vi "Interpolate_Calib_Coeff.vi"(5 "Analysis Info cluster":T1={"Colour"=0, "Inst type"=enum."Pitot-static tube", "Inst name"="Manometer voltage", "Symbol"="U", "Code name"="", "Extra Info"="U", "Inst Array"=enum."PWA", "Extra Titles"=[], "Extra Values"=[], "U"=0.0, "u^2"=0.0, "u^3"=0.0, "u^4"=0.0, "Skew_u"=0.0, "Kurt_u"=0.0, "Sd Error in Mean"=0.0, "% u'/U"=0.0, "X"=0.0, "Y"=0.0, "Z"=0.0, "Timescale integral to 25%"=0.0, "Sd Error in Variance"=0.0, "Calib File"=path "", "Calib Constants"=[], "Output Position"=FALSE, "Full Stats"=FALSE, "Av Sampling Rate"=0.0, "Av No of Samples"=0.0, "Total Meas Time (s)"=0.0, "ADAM Ch Name"=""} {"Sd Error in Variance" format="%.2f"; "Skew_u" format="%.2f"; "% u'/U" format="%.2f"; "Sd Error in Mean" format="%.2f"; "Kurt_u" format="%.2f"; "u^4" format="%.2f"; "u^3" format="%.2f"; "U" format="%.2f"; "u^2" format="%.2f"}, 7 "Take New Data?":bool) -> (0 "Calib Coeff":dbl[](array[numeric]), 1 "Calib Type Name":string, 2 "Calib file string":string, 3 "Read file":bool, 4 "Analysis Info cluster  Out":T1={"Colour"=0, "Inst type"=enum."Pitot-static tube", "Inst name"="Manometer voltage", "Symbol"="U", "Code name"="", "Extra Info"="U", "Inst Array"=enum."PWA", "Extra Titles"=[], "Extra Values"=[], "U"=0.0, "u^2"=0.0, "u^3"=0.0, "u^4"=0.0, "Skew_u"=0.0, "Kurt_u"=0.0, "Sd Error in Mean"=0.0, "% u'/U"=0.0, "X"=0.0, "Y"=0.0, "Z"=0.0, "Timescale integral to 25%"=0.0, "Sd Error in Variance"=0.0, "Calib File"=path "", "Calib Constants"=[], "Output Position"=FALSE, "Full Stats"=FALSE, "Av Sampling Rate"=0.0, "Av No of Samples"=0.0, "Total Meas Time (s)"=0.0, "ADAM Ch Name"=""} {"Sd Error in Variance" format="%.2f"; "Skew_u" format="%.2f"; "% u'/U" format="%.2f"; "Sd Error in Mean" format="%.2f"; "Kurt_u" format="%.2f"; "u^4" format="%.2f"; "u^3" format="%.2f"; "U" format="%.2f"; "u^2" format="%.2f"})   [LabVIEW 2012]
uses:
  Controls/Analysis_info_cluster.ctl
  Controls/Inst_type.ctl
  Controls/Instrument_Array.ctl
  XW calib map/Map method.ctl
  Globals/Meas_global.vi
  XW calib map/XW_Map_Global.vi
  Globals/Plug_in_data_global.vi
  <vilib>/Analysis/NI_AALPro.lvlib
panel:
  in  "TAKE NEW DATA XW Map method":T4=enum."Const. Psi_eff (std.)"
  in  "Domain padding factor":dbl=1.01
  in  "cap indicial sum to n":bool=TRUE
  in  "surface order (n)":i32=5
  in  "Apply calibration corrections":bool=TRUE
  in  "POST PROC. XW Map method":T4=enum."Psi_eff, k = f(Umagn.)"
  in  "variable n":bool=TRUE
  in  "wire diameter (mu.m)":dbl=5.0
  out "Header info":string[][](array[string])
  # "For polysurface method only:"
  # "For trimesh method only"
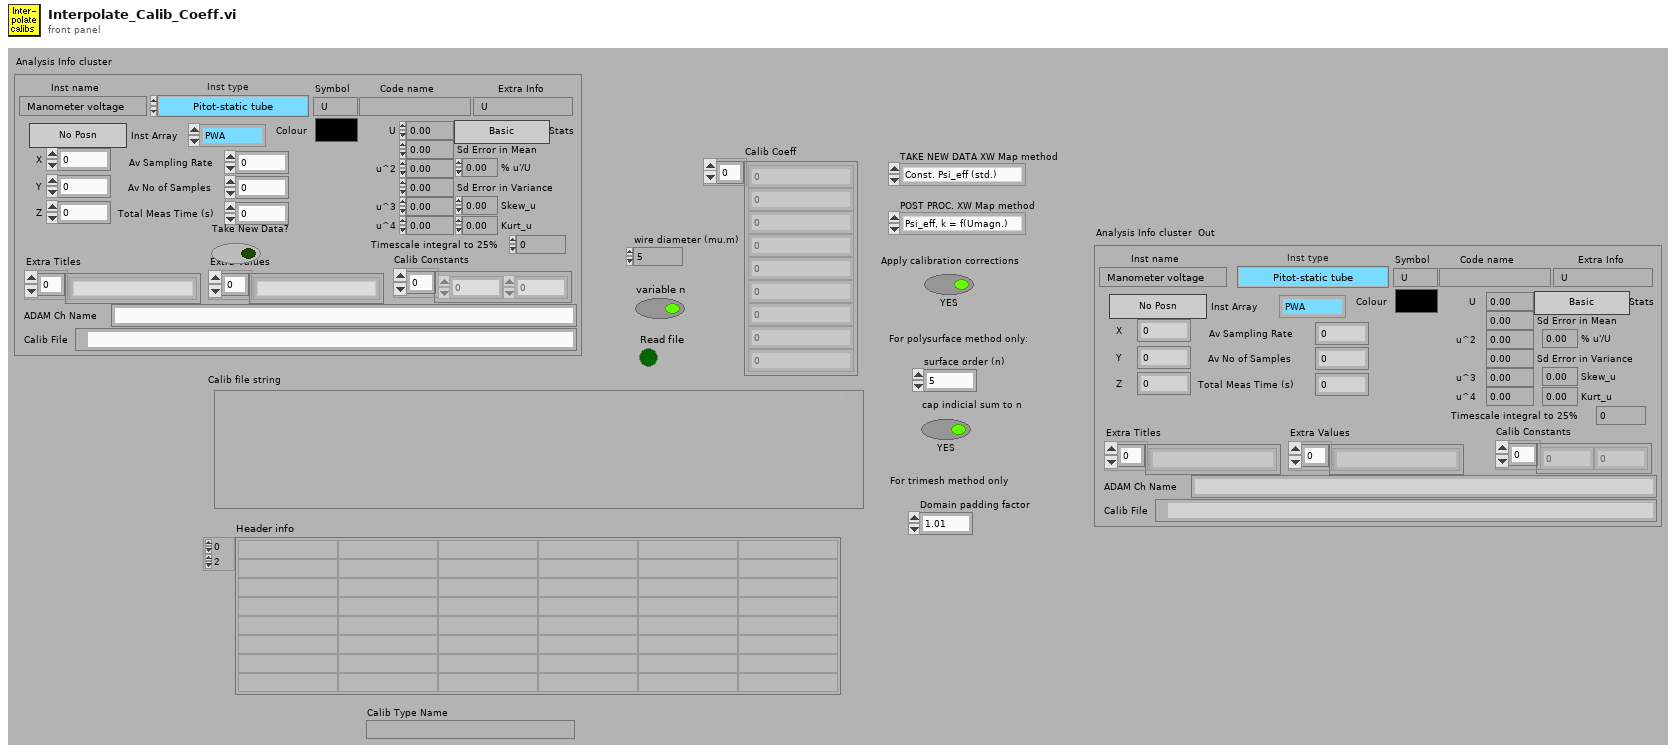
[diagram p1: front panel]
types:
  T1 = typedef "Analysis_info_cluster.ctl" = cluster{"Colour":u32, "Inst type":T2, "Inst name":string, "Symbol":string, "Code name":string, "Extra Info":string, "Inst Array":T3, "Extra Titles":string[], "Extra Values":string[], "U":dbl, "u^2":dbl, "u^3":dbl, "u^4":dbl, "Skew_u":dbl, "Kurt_u":dbl, "Sd Error in Mean":dbl, "% u'/U":dbl, "X":dbl, "Y":dbl, "Z":dbl, "Timescale integral to 25%":dbl, "Sd Error in Variance":dbl, "Calib File":path, "Calib Constants":dbl[], "Output Position":bool, "Full Stats":bool, "Av Sampling Rate":dbl, "Av No of Samples":dbl, "Total Meas Time (s)":dbl, "ADAM Ch Name":string}
  T2 = typedef "Inst_type.ctl" = enum16{"Propeller anemometer", "Raw voltage", "Pressure Transducer", "Pitot-static tube", "Preston tube", "Hot wire", "Cross wire 1", "Cross wire 2", "Generic Linear", "Generic Polynomial", "Generic BackPoly", "Fast FID", "Thermocouple", "Cold wire", "Pulsed Wire", "LDA Vel", "LDA Tran time", "LDA Arr time"}
  T3 = typedef "Instrument_Array.ctl" = enum16{"PWA", "LDA", "Analogue"}
  T4 = typedef "Map method.ctl" = enum16{"Triangle mesh", "Polynomial surface", "Const. Psi_eff (std.)", "Psi_eff = f(Umagn.)", "Psi_eff, k = f(Umagn.)"}
  T5 = cluster{"1st Calib time":dbl, "2nd Calib time":dbl, "Meas start time":dbl, "Meas end time":dbl, "Fraction":dbl}
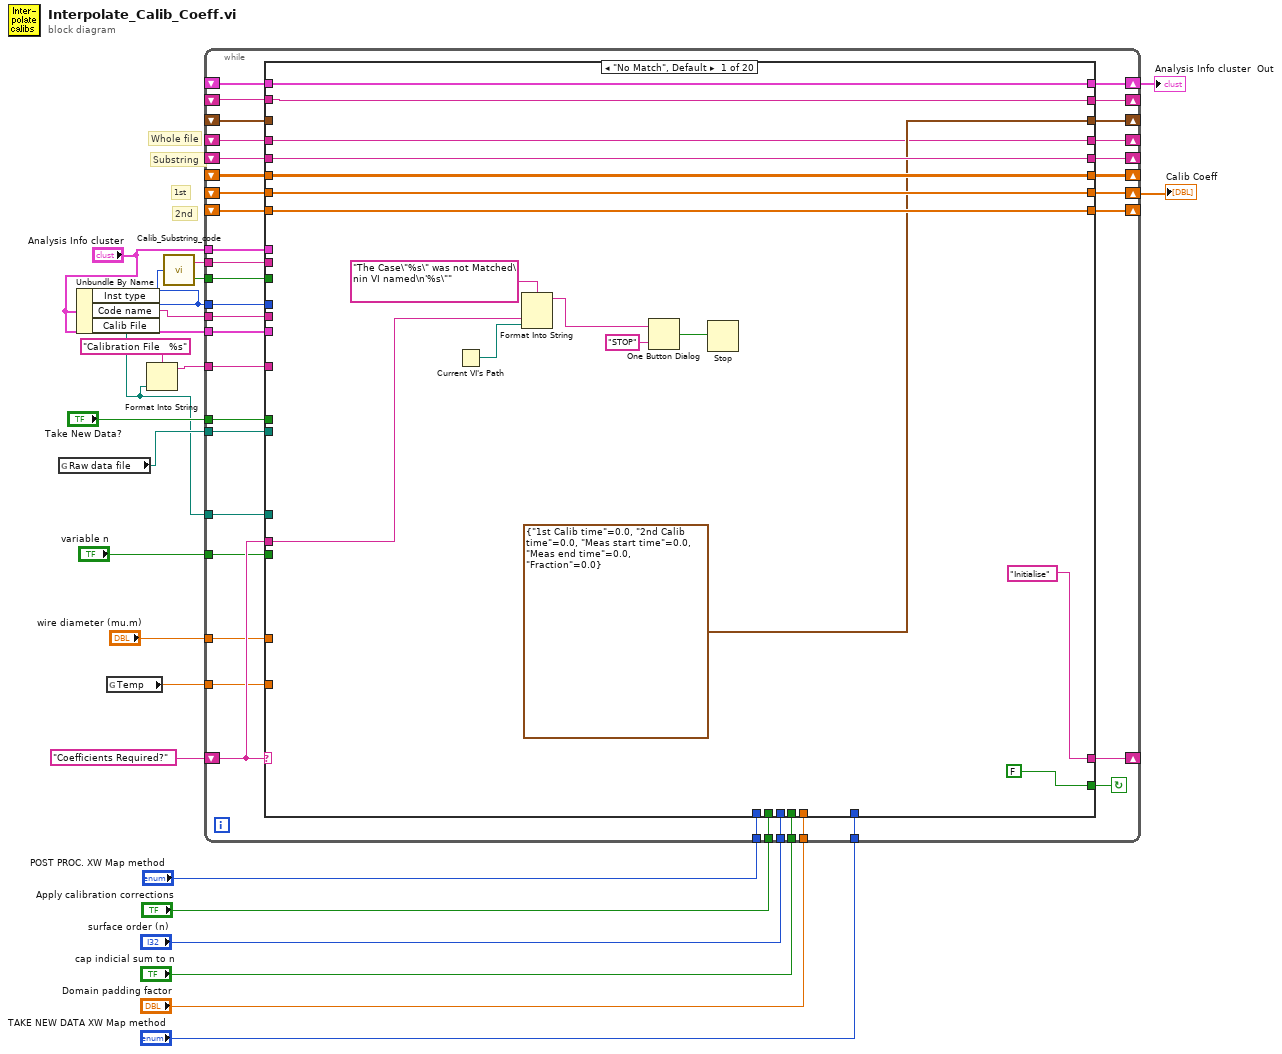
[diagram p0: block diagram]
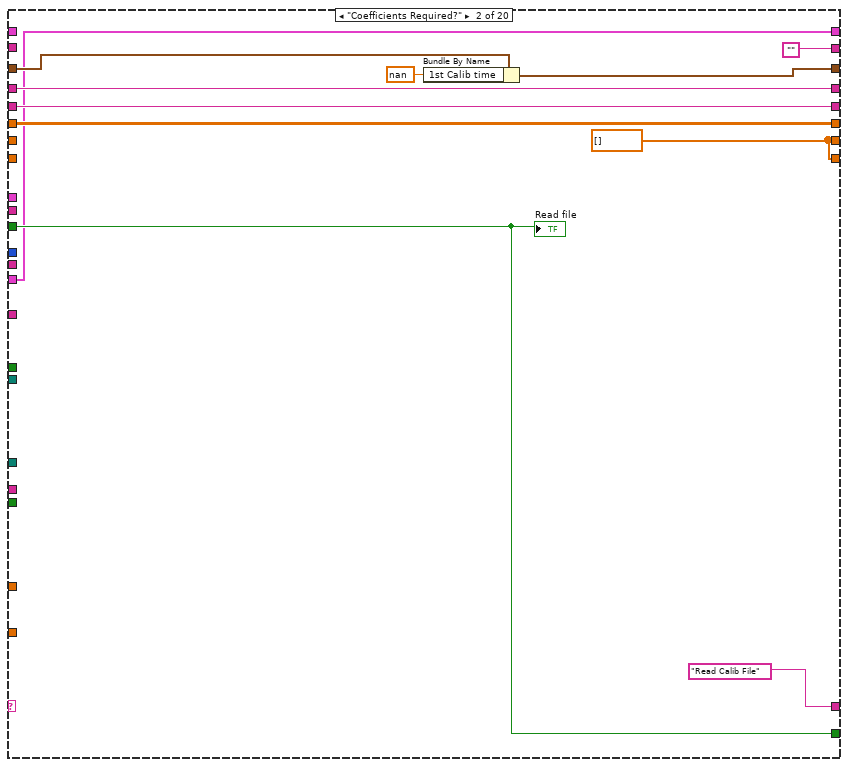
[diagram p2: hidden frame]
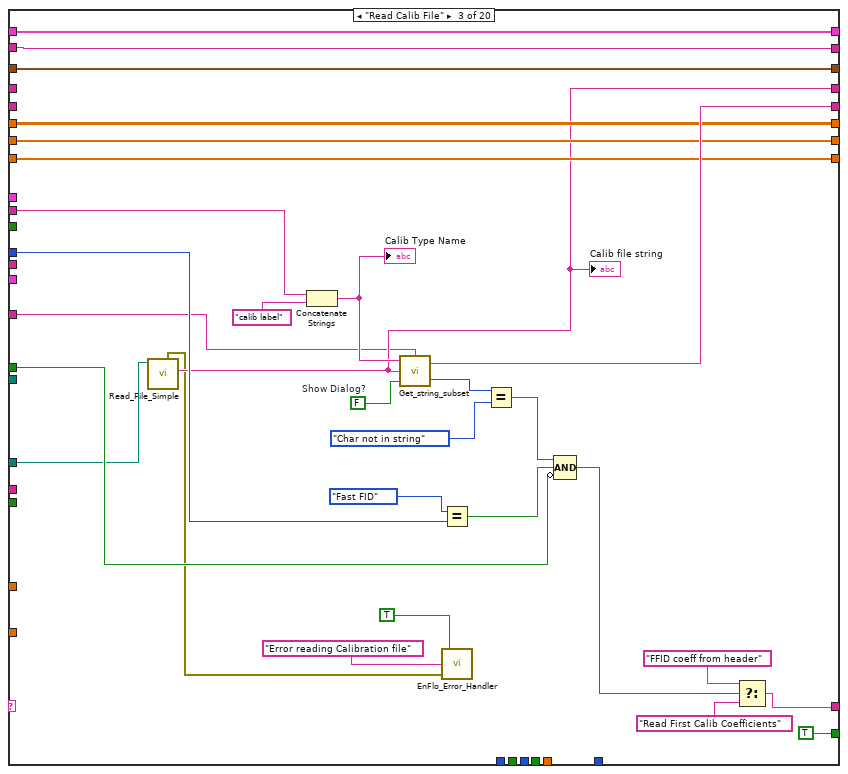
[diagram p3: hidden frame]
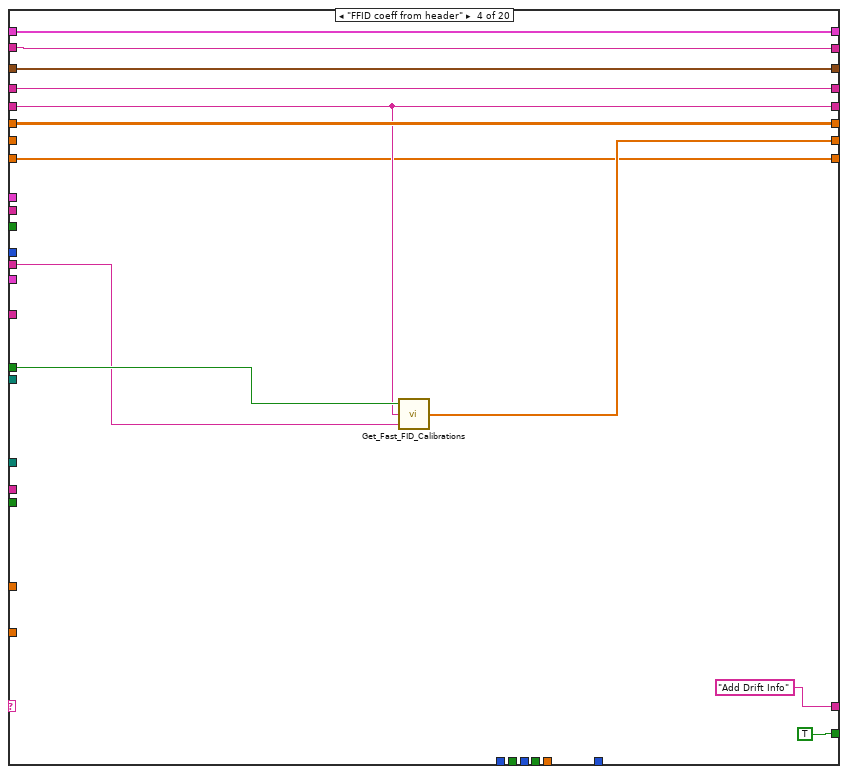
[diagram p4: hidden frame]
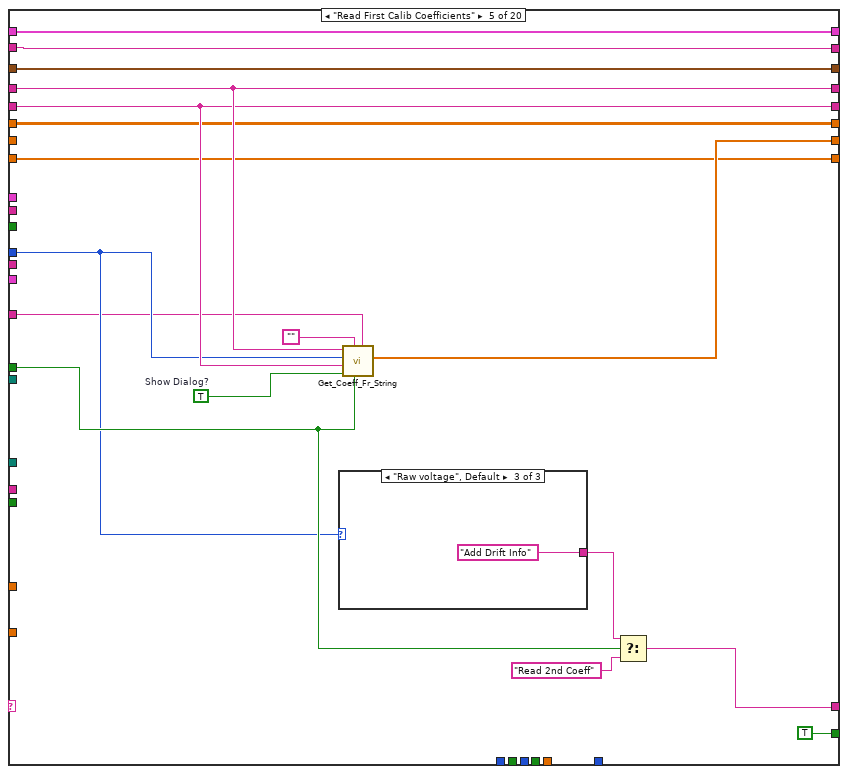
[diagram p5: hidden frame]
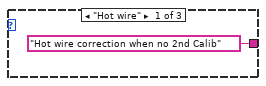
[diagram p6: hidden frame]
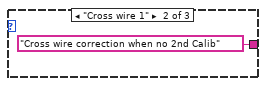
[diagram p7: hidden frame]
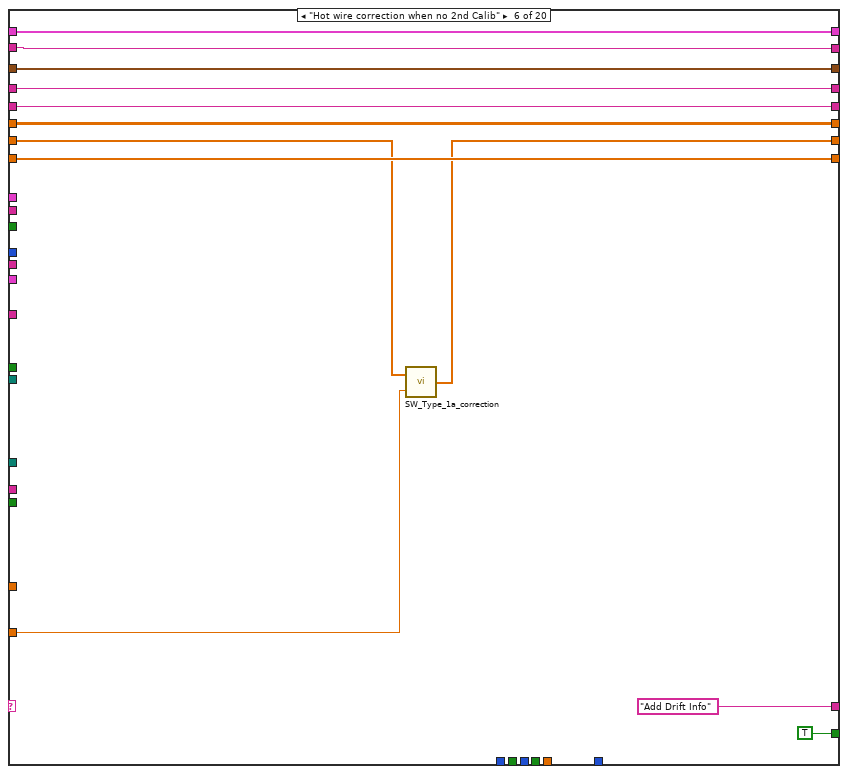
[diagram p8: hidden frame]
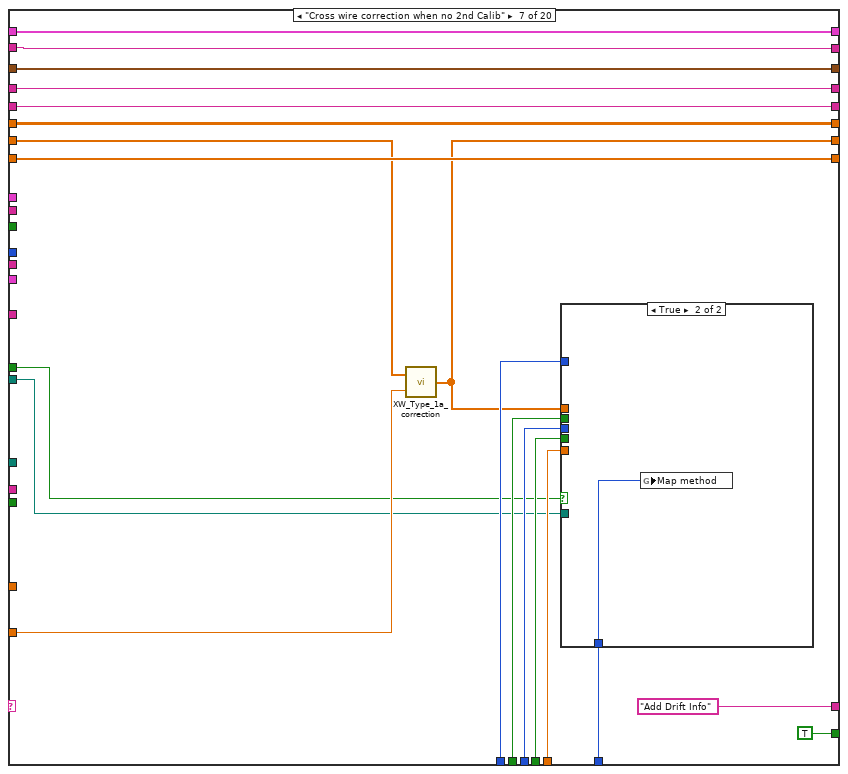
[diagram p9: hidden frame]
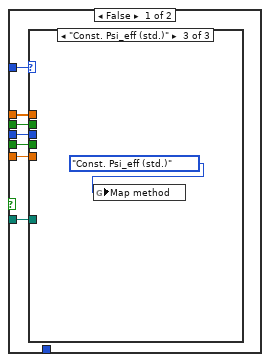
[diagram p10: hidden frame]
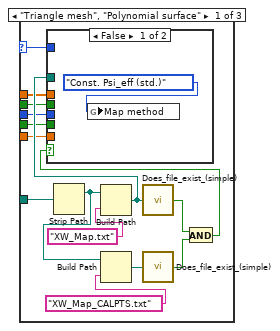
[diagram p11: hidden frame]
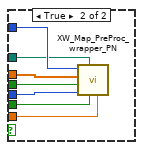
[diagram p12: hidden frame]
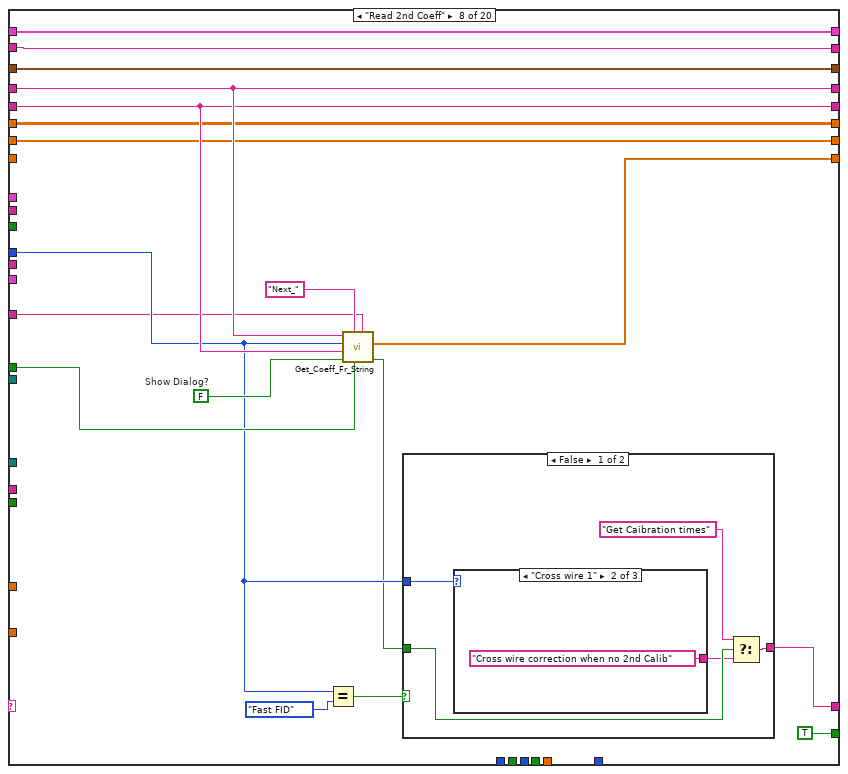
[diagram p14: hidden frame]
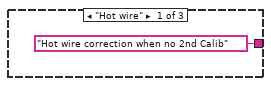
[diagram p15: hidden frame]
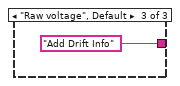
[diagram p16: hidden frame]
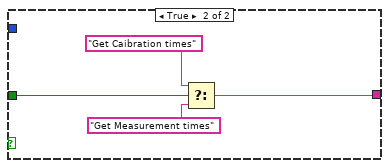
[diagram p17: hidden frame]
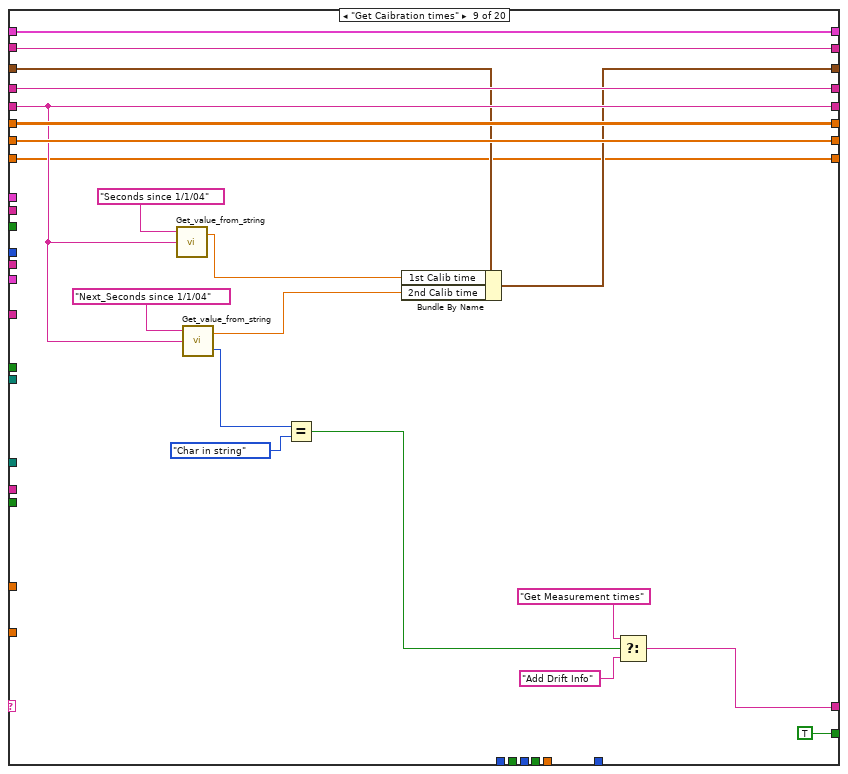
[diagram p18: hidden frame]
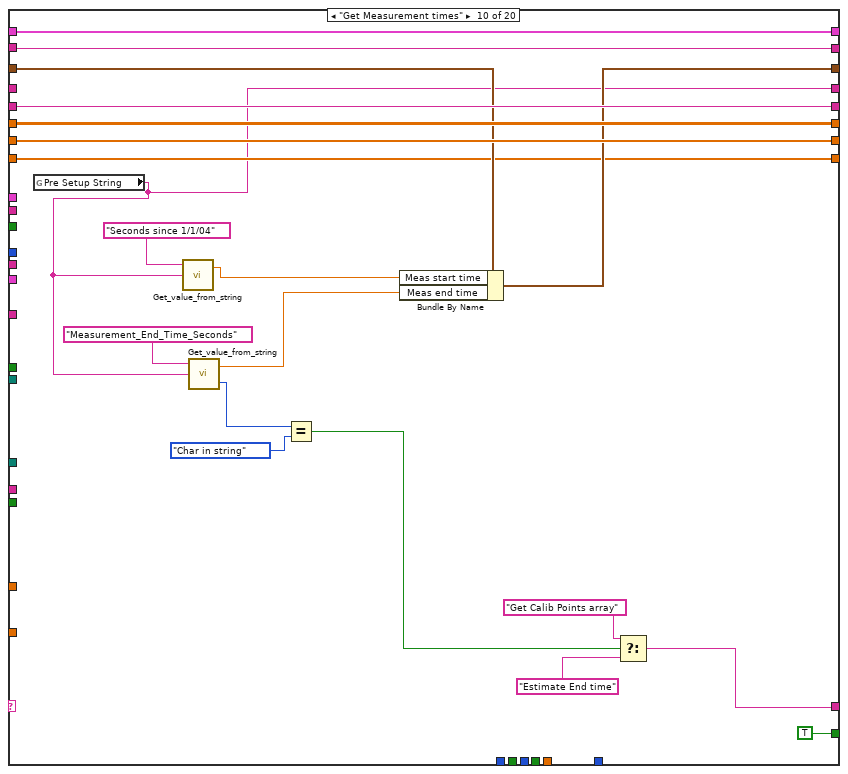
[diagram p19: hidden frame]
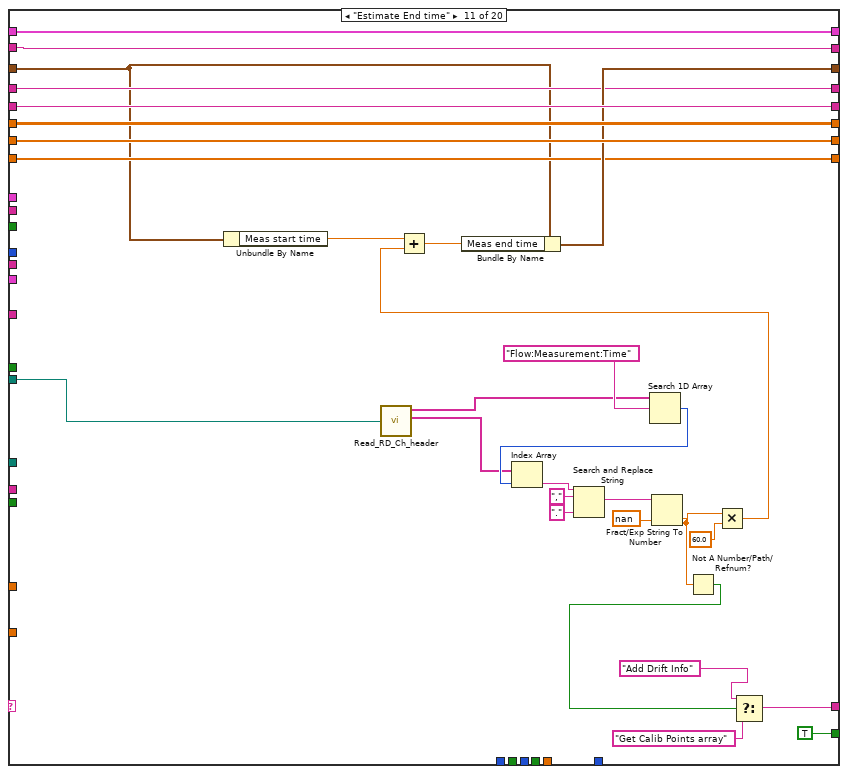
[diagram p20: hidden frame]
diagram:
  # "Substring"
  # "2nd"
  # "Whole file"
  # "1st"
  n1 = global read "Meas_global.vi" "Raw data file"() -> (w15:path)
  n2 = Unbundle By Name("Analysis Info cluster") -> ("Inst type"=w18:T2, "Code name"=w19:string, "Calib File"=w1:path)
  n3 = global read "Meas_global.vi" "Temp"() -> (w14:dbl)
  n4 = Format Into String(format string="Calibration File   %s", w1) -> (resulting string=w2:string)  [unwired: 2 in, 1 out]
  n5 = call "Calib_Substring_code.vi"("Inst type"=w18) -> ("Substring Type"=w16:string, "Read file"=w17:bool)
  n6 = while {
    tunnel: w1 -> [w51]
    shift-left: _ -> [w52]
    shift-right: [w53] -> _
    shift-left: _ -> [w54]
    shift-right: [w56] -> w21
    tunnel: w18 -> [w58]
    shift-left: _ -> [w55]
    shift-right: [w57] -> _
    shift-left: "Coefficients Required?" -> [w59]
    shift-right: [w24] -> _
    tunnel: "Take New Data?" -> [w50]
    tunnel: w19 -> [w49]
    shift-right: [w48] -> _
    shift-left: _ -> [w47]
    shift-right: [w46] -> _
    shift-left: _ -> [w45]
    shift-right: [w44] -> _
    shift-left: _ -> [w43]
    tunnel: w17 -> [w42]
    tunnel: w16 -> [w41]
    tunnel: w15 -> [w40]
    shift-right: [w39] -> _
    shift-left: _ -> [w38]
    tunnel: w14 -> [w37]
    tunnel: "wire diameter (mu.m)" -> [w36]
    tunnel: "variable n" -> [w35]
    tunnel: "POST PROC. XW Map method" -> [w34]
    tunnel: "Apply calibration corrections" -> [w33]
    tunnel: "surface order (n)" -> [w32]
    tunnel: "cap indicial sum to n" -> [w31]
    tunnel: "Domain padding factor" -> [w30]
    tunnel: "TAKE NEW DATA XW Map method" -> [w29]
    tunnel: "Analysis Info cluster" -> [w28]
    shift-right: [w26] -> w5
    shift-left: _ -> [w27]
    tunnel: "Analysis Info cluster" -> [w25]
    tunnel: w2 -> [w23]
    stop <- w60 continue-if-true
    n7 = case shown="\"No Match\", Default" w59 {
      tunnel: [FALSE w82 TRUE ("Read file") TRUE TRUE ("Read file") TRUE ("Read file") TRUE ("Read file") TRUE ("Read file") TRUE ("Read file") TRUE ("Read file") TRUE ("Read file") TRUE ("Read file") TRUE ("Read file") TRUE ("Read file") TRUE ("Read file") TRUE ("Read file") w510 w701 TRUE ("Read file") FALSE ("Read file")] -> w60
      tunnel: ["Initialise" "Read Calib File" w102 "Add Drift Info" w132 "Add Drift Info" "Add Drift Info" w224 w259 w280 w294 w329 "FFID Bkgnd correction method" ("f") "Add Drift Info" ("f") "Add Drift Info" ("f") w495 w511 w702 "Add Drift Info" "End"] -> w24
      tunnel: w59 -> [w71 _ _ _ _ _ _ _ _ _ _ _ _ _ _ _ _ _ _ _]
      tunnel: w58 -> [_ _ w109 _ w134 _ _ w216 _ _ _ w315 _ _ _ _ _ _ _ _]
      tunnel: [w68 w86 w115 w124 w142 w159 w179 w228 w253 w274 w308 w333 w368 w401 w447 w505 w518 w709 w809 w838] -> w57
      tunnel: [w67 w84 w99 w122 w144 w151 w162 w222 w258 w279 w309 w332 w358 w400 w407 w493 w514 w705 w800 w832] -> w56
      tunnel: w55 -> [w68 w86 _ w124 w142 w159 w179 w228 w253 w274 w308 w333 w368 w401 w447 w505 w519 w710 w809 w838]
      tunnel: w54 -> [w67 _ w99 _ _ w152 w170 w222 w258 w279 w309 w332 w359 w387 w431 w493 w515 w706 w801 w847]
      tunnel: [w66 w85 w114 w128 w141 w158 w178 w227 w261 w282 w311 w331 w354 w383 w421 w501 w517 w708 w805 w856] -> w53
      tunnel: w52 -> [w66 w85 w114 w128 w141 w158 w178 w227 w261 w282 w311 _ w354 w383 w421 w501 w516 w707 w805 w856]
      tunnel: w51 -> [_ _ w89 _ _ _ _ _ _ _ _ _ _ _ _ _ _ _ _ _]
      tunnel: w50 -> [_ _ w105 w125 w138 _ w165 w225 _ _ _ _ _ _ w409 _ _ _ _ w830]
      tunnel: w49 -> [_ _ _ w123 _ _ _ _ _ _ _ _ _ _ _ _ w522 w713 _ _]
      tunnel: [w65 w84 w98 w121 w140 w157 w177 w221 w245 w266 w306 w316 w361 w386 w432 w504 w513 w704 w808 w855] -> w48
      tunnel: w47 -> [w65 _ w98 w121 w140 w157 w177 _ w245 w266 w306 w316 w361 w386 w432 w504 w512 w703 w808 w855]
      tunnel: [w63 w83 w97 w119 w143 w160 w180 w229 w262 w265 w305 w328 w355 w397 w444 w502 w520 w711 w806 w857] -> w46
      tunnel: w45 -> [w63 w83 _ w119 w143 w160 w180 w229 w262 _ w305 w328 w355 w397 w444 w502 w523 w714 w806 w857]
      tunnel: [T5 {"1st Calib time"=0.0, "2nd Calib time"=0.0, "Meas start time"=0.0, "Meas end time"=0.0, "Fraction"=0.0} w80 w96 w120 w137 w155 w175 w220 w249 w270 w307 w317 w356 w398 w445 w503 w509 w700 w807 w835] -> w44
      tunnel: w43 -> [_ w81 w96 w120 w137 w155 w175 w220 w252 w273 w304 w319 w356 w398 w445 w503 w521 w712 w807 w835]
      tunnel: w42 -> [_ w82 _ _ _ _ _ _ _ _ _ _ _ _ _ _ _ _ _ _]
      tunnel: w41 -> [_ _ w95 _ _ _ _ _ _ _ _ _ _ _ _ _ _ _ _ _]
      tunnel: w40 -> [_ _ _ _ _ _ w164 _ _ _ w292 _ _ _ w410 w494 _ _ _ w831]
      tunnel: [w62 "" w94 w118 w135 w154 w174 w217 w244 w264 w293 w313 w345 w389 w436 w492 w508 w698 w797 w834] -> w39
      tunnel: w38 -> [w62 _ w94 w118 w135 w154 w174 w217 w244 w264 w293 w313 w347 w391 w438 w492 w507 w699 w798 w834]
      tunnel: w37 -> [_ _ _ _ _ w150 w172 _ _ _ _ _ _ w378 w412 _ _ _ _ _]
      tunnel: w36 -> [_ _ _ _ _ _ _ _ _ _ _ _ _ w376 w411 _ _ _ _ _]
      tunnel: w35 -> [_ _ _ _ _ _ _ _ _ _ _ _ _ w377 w413 _ _ _ _ _]
      tunnel: w34 -> [_ _ _ _ _ _ w171 _ _ _ _ _ _ _ w408 _ _ _ _ w829]
      tunnel: w33 -> [_ _ _ _ _ _ w169 _ _ _ _ _ _ _ w406 _ _ _ _ _]
      tunnel: w32 -> [_ _ _ _ _ _ w168 _ _ _ _ _ _ _ w405 _ _ _ _ _]
      tunnel: w31 -> [_ _ _ _ _ _ w167 _ _ _ _ _ _ _ w404 _ _ _ _ _]
      tunnel: w30 -> [_ _ _ _ _ _ w166 _ _ _ _ _ _ _ w403 _ _ _ _ _]
      tunnel: w29 -> [_ _ _ _ _ _ w163 _ _ _ _ _ _ _ _ _ _ _ _ _]
      tunnel: w28 -> [_ w77 _ _ _ _ _ _ _ _ _ _ _ _ _ _ _ _ _ w828]
      tunnel: w27 -> [w61 _ w90 w117 w131 w149 w161 w214 w243 w263 w289 w312 w344 w375 w402 w491 w506 w697 w796 _]
      tunnel: [w61 w77 w90 w117 w131 w149 w161 w214 w243 w263 w289 w312 w344 w375 w402 w491 w506 w697 w796 w827] -> w26
      tunnel: w25 -> [_ _ _ _ _ _ _ _ _ _ _ _ _ _ _ _ _ _ _ _]
      tunnel: w23 -> [_ _ w88 _ w130 _ _ w213 _ _ _ _ _ _ _ _ _ _ _ _]
      frame "No Match", Default {
        n8 = Current VI's Path() -> (path=w70:path)
        n9 = Format Into String(format string="The Case\"%s\" was not Matched\nin VI named\n'%s\"" ("Format String"), w71, w70) -> (resulting string=w74:string)  [unwired: 2 in, 1 out]
        n10 = One Button Dialog(message=w74, button name ("OK")="STOP") -> (true=w72:bool)
        n11 = Stop(stop? (T)=w72) -> ()
      }
      frame "Coefficients Required?" {
        w84 = dbl[] [] ("Calib Coeff")
        n12 = Bundle By Name(cluster=w81, "1st Calib time"=nan) -> (w80:T5)
        "Read file" <- w82
      }
      frame "Read Calib File" {
        w110 = FALSE  # Show Dialog?
        n13 = call "Read_File_Simple.vi"("Filename"=w89) -> ("error out"=w93:errorcluster, "string"=w97:string)  [unwired: 2 in, 6 out]
        "Calib file string" <- w97
        n14 = Concatenate Strings(w95, "calib label") -> (w113:string)
        "Calib Type Name" <- w113
        n15 = call "Get_string_subset.vi"("String Name"=w88, "Show Dialog?"=w110, "String to split"=w97, "File Label"=w113) -> ("Status"=w112:enum16{"Char in string", "Char not in string"}, "Output string"=w115:string)
        n16 = Equal?(x=Inst_type."Fast FID" ("Inst type"), y=w109) -> (x = y?=w106:bool)
        n17 = call "EnFlo_Error_Handler.vi"("error in (no error)"=w93, "Error Type"="Error reading Calibration file", "Dialog Box (T)"=TRUE) -> ()  [unwired: 3 out]
        n18 = Equal?(x=w112, y=enum16{"Char in string", "Char not in string"}."Char not in string" ("Status")) -> (x = y?=w107:bool)
        n19 = Compound Arithmetic op=AND(w107, w106, invert w105) -> (w103:bool)
        n20 = Select(t="FFID coeff from header", s=w103, f="Read First Calib Coefficients") -> (s? t:f=w102:string)
      }
      frame "FFID coeff from header" {
        n21 = call "Get_Fast_FID_Calibrations.vi"("Code Name"=w123, "Calib File String"=w124, "Take New Data"=w125) -> ("Calib Constants"=w122:dbl[])
      }
      frame "Read First Calib Coefficients" {
        w145 = TRUE  # Show Dialog?
        n22 = case shown="\"Raw voltage\", Default" w134 {
          tunnel: ["Hot wire correction when no 2nd Calib" "Cross wire correction when no 2nd Calib" "Add Drift Info"] -> w133
          frame "Hot wire" {
          }
          frame "Cross wire 1" {
          }
          frame "Raw voltage", Default {
          }
        }
        n23 = call "Get_Coeff_Fr_String.vi"("String Name"=w130, "Take New Data?"=w138, "Prefix"="", "Show Dialog?"=w145, "Sub String"=w142, "Inst type"=w134, "Whole String"=w143) -> ("Calib Constants"=w144:dbl[])  [unwired: 2 in, 1 out]
        n24 = Select(t=w133, s=w138, f="Read 2nd Coeff") -> (s? t:f=w132:string)
      }
      frame "Hot wire correction when no 2nd Calib" {
        n25 = call "SW_Type_1a_correction.vi"("Tmeas (degC)"=w150, "Calib consts."=w152) -> ("Corrected calib consts."=w151:dbl[])
      }
      frame "Cross wire correction when no 2nd Calib" {
        n26 = call "XW_Type_1a_correction.vi"("Tmeas (degC)"=w172, "Calib consts."=w170) -> ("Corrected calib consts."=w162:dbl[])
        n27 = case shown="True" w165 {
          tunnel: w164 -> [w187 _]
          tunnel: w171 -> [w181 _]
          tunnel: w162 -> [w186 _]
          tunnel: w169 -> [w185 _]
          tunnel: w168 -> [w184 _]
          tunnel: w167 -> [w183 _]
          tunnel: w166 -> [w182 _]
          tunnel: w163 -> [_ w212]
          frame False {
            n28 = case shown="\"Const. Psi_eff (std.)\"" w181 {
              selector: w181 -> [w194 _ _]
              tunnel: w187 -> [w202 _ _]
              tunnel: w186 -> [w199 _ _]
              tunnel: w185 -> [w198 _ _]
              tunnel: w184 -> [w197 _ _]
              tunnel: w183 -> [w196 _ _]
              tunnel: w182 -> [w195 _ _]
              frame "Triangle mesh", "Polynomial surface" {
                n29 = Strip Path(path=w202) -> (stripped path=w191:path)  [unwired: 1 out]
                n30 = Build Path(base path=w191, name or relative path="XW_Map.txt") -> (appended path=w200:path)
                n31 = Build Path(base path=w191, name or relative path="XW_Map_CALPTS.txt") -> (appended path=w193:path)
                n32 = call "Does_file_exist_(simple).vi"("Pathname"=w200) -> ("exists?"=w189:bool)
                n33 = call "Does_file_exist_(simple).vi"("Pathname"=w193) -> ("exists?"=w190:bool)
                n34 = And(x=w189, y=w190) -> (x .and. y?=w188:bool)
                n35 = case shown="False" w188 {
                  tunnel: w200 -> [_ w209]
                  tunnel: w194 -> [_ w210]
                  tunnel: w199 -> [_ w208]
                  tunnel: w198 -> [_ w207]
                  tunnel: w197 -> [_ w206]
                  tunnel: w196 -> [_ w205]
                  tunnel: w195 -> [_ w204]
                  frame False {
                    n36 = global write "XW_Map_Global.vi" "Map method"(Map_method."Const. Psi_eff (std.)" ("Map method")) -> ()
                  }
                  frame True {
                    n37 = call "XW_Map_PreProc_wrapper_PN.vi"("Domain padding factor"=w204, "cap indicial sum to n"=w205, "XW_Calib_Map file path"=w209, "surface order (n)"=w206, "Apply calibration corrections"=w207, "Calib const"=w208, "Map method"=w210) -> ()  [unwired: 5 out]
                  }
                }
              }
              frame "Psi_eff = f(Umagn.)", "Psi_eff, k = f(Umagn.)" {
              }
              frame "Const. Psi_eff (std.)" {
                n38 = global write "XW_Map_Global.vi" "Map method"(Map_method."Const. Psi_eff (std.)" ("Map method")) -> ()
              }
            }
          }
          frame True {
            n39 = global write "XW_Map_Global.vi" "Map method"(w212) -> ()
          }
        }
      }
      frame "Read 2nd Coeff" {
        w230 = FALSE  # Show Dialog?
        n40 = Equal?(x=w216, y=Inst_type."Fast FID" ("Inst type")) -> (x = y?=w218:bool)
        n41 = call "Get_Coeff_Fr_String.vi"("String Name"=w213, "Take New Data?"=w225, "Prefix"="Next_", "Show Dialog?"=w230, "Sub String"=w228, "Inst type"=w216, "Whole String"=w229) -> ("Coefficients Found?"=w215:bool, "Calib Constants"=w221:dbl[])  [unwired: 2 in]
        n42 = case shown="False" w218 {
          tunnel: [w231 w242] -> w224
          tunnel: w215 -> [w233 w239]
          tunnel: w216 -> [w235 _]
          frame False {
            n43 = case shown="\"Cross wire 1\"" w235 {
              tunnel: ["Hot wire correction when no 2nd Calib" "Cross wire correction when no 2nd Calib" "Add Drift Info"] -> w232
              frame "Hot wire" {
              }
              frame "Cross wire 1" {
              }
              frame "Raw voltage", Default {
              }
            }
            n44 = Select(t="Get Caibration times", s=w233, f=w232) -> (s? t:f=w231:string)
          }
          frame True {
            n45 = Select(t="Get Caibration times", s=w239, f="Get Measurement times") -> (s? t:f=w242:string)
          }
        }
      }
      frame "Get Caibration times" {
        n46 = call "Get_value_from_string.vi"("Input string"=w253, "Variable name"="Seconds since 1/1/04") -> ("Value"=w251:dbl)  [unwired: 1 in, 1 out]
        n47 = call "Get_value_from_string.vi"("Input string"=w253, "Variable name"="Next_Seconds since 1/1/04") -> ("Status"=w248:enum16{"Char in string", "Char not in string"}, "Value"=w250:dbl)  [unwired: 1 in]
        n48 = Equal?(x=w248, y=enum16{"Char in string", "Char not in string"}."Char in string" ("Status")) -> (x = y?=w246:bool)
        n49 = Bundle By Name(cluster=w252, "1st Calib time"=w251, "2nd Calib time"=w250) -> (w249:T5)
        n50 = Select(t="Get Measurement times", s=w246, f="Add Drift Info") -> (s? t:f=w259:string)
      }
      frame "Get Measurement times" {
        n51 = global read "Meas_global.vi" "Pre Setup String"() -> (w265:string)
        n52 = call "Get_value_from_string.vi"("Input string"=w265, "Variable name"="Seconds since 1/1/04") -> ("Value"=w272:dbl)  [unwired: 1 in, 1 out]
        n53 = call "Get_value_from_string.vi"("Input string"=w265, "Variable name"="Measurement_End_Time_Seconds") -> ("Status"=w269:enum16{"Char in string", "Char not in string"}, "Value"=w271:dbl)  [unwired: 1 in]
        n54 = Equal?(x=w269, y=enum16{"Char in string", "Char not in string"}."Char in string" ("Status")) -> (x = y?=w267:bool)
        n55 = Bundle By Name(cluster=w273, "Meas start time"=w272, "Meas end time"=w271) -> (w270:T5)
        n56 = Select(t="Get Calib Points array", s=w267, f="Estimate End time") -> (s? t:f=w280:string)
      }
      frame "Estimate End time" {
        n57 = Unbundle By Name(w304) -> ("Meas start time"=w303:dbl)
        n58 = call "Read_RD_Ch_header.vi"("Raw data file"=w292) -> ("Ch Name Out"=w291:string[], "Ch Values"=w290:string[])  [unwired: 2 out]
        n59 = Search 1D Array(1D array=w291, element="Flow:Measurement:Time") -> (index of element=w300:i32)  [unwired: 1 out]
        n60 = Index Array(array=w290, index=w300) -> (element=w285:string)
        n61 = Search and Replace String(input string=w285, search string=",", replace string="." ("replace string (\"\")")) -> (result string=w286:string)  [unwired: 5 in, 3 out]
        n62 = Fract/Exp String To Number(string=w286, default (0 dbl)=nan ("default (0 DBL)")) -> (number=w283:dbl)  [unwired: 3 out]
        n63 = Not A Number/Path/Refnum?(number/path/refnum=w283) -> (NaN/Path/Refnum?=w297:bool)
        n64 = Multiply(x=w283, y=60.0) -> (x*y=w298:dbl)
        n65 = Add(x=w303, y=w298) -> (x+y=w302:dbl)
        n66 = Bundle By Name(cluster=w304, "Meas end time"=w302) -> (w307:T5)
        n67 = Select(t="Add Drift Info", s=w297, f="Get Calib Points array") -> (s? t:f=w294:string)
      }
      frame "Get Calib Points array" {
        w335 = FALSE  # Show Dialog?
        # "Fraction = (Av_Meas_Time - Calib1_time)  /  (Calib2_time - Calib1_time)"
        n68 = Unbundle By Name(w319) -> ("Meas start time"=w324:dbl, "Meas end time"=w323:dbl, "2nd Calib time"=w325:dbl, "1st Calib time"=w314:dbl)
        n69 = Add(x=w324, y=w323) -> (x+y=w327:dbl)
        n70 = call "2D_array_from_string.vi"("Show Dialog?"=w335, "Input string"=w333, "Array title"="Calib points label") -> ("2D data array"=w331:dbl[][])  [unwired: 1 in]
        n71 = Divide(x=w327, y=2.0) -> (x/y=w322:dbl)
        n72 = Subtract(x=w325, y=w314) -> (x-y=w320:dbl)
        n73 = Subtract(x=w322, y=w314) -> (x-y=w321:dbl)
        n74 = Divide(x=w321, y=w320) -> (x/y=w318:dbl)
        n75 = case shown="\"Hot wire\"" w315 {
          tunnel: ["Add Drift Info" "Single Hot wire" "Cross wire" w340] -> w329
          tunnel: w314 -> [_ _ _ w343]
          frame "Propeller anemometer", Default {
          }
          frame "Hot wire" {
          }
          frame "Cross wire 1" {
          }
          frame "Fast FID" {
            n76 = Not A Number/Path/Refnum?(number/path/refnum=w343) -> (NaN/Path/Refnum?=w342:bool)
            n77 = Select(t="FFID Bkgnd correction method", s=w342, f="Fast FID") -> (s? t:f=w340:string)
          }
        }
        n78 = Bundle By Name(cluster=w319, "Fraction"=w318) -> (w317:T5)
      }
      frame "Fast FID" {
        # "Concentrations"
        # "Voltage"
        # "End"
        # "Start"
        # "(End-Start)*Fraction + Start"
        n79 = Index Array(array=w354, index (col)=1) -> (element=w364:dbl[])  [unwired: 1 in]
        n80 = call "2nd_order_Poly_convert.vi"("Calib constants"=w361, "Voltage"=w364) -> ("Eng Values"=w365:dbl[])  [unwired: 4 out]
        n81 = call "2nd_order_Poly_convert.vi"("Calib constants"=w359, "Voltage"=w364) -> ("Eng Values"=w366:dbl[])  [unwired: 4 out]
        n82 = Unbundle By Name(w356) -> ("Fraction"=w351:dbl)
        n83 = In Range and Coerce(upper limit=1.0, x=w351, lower limit=0.0) -> (coerced(x)=w348:dbl)  [unwired: 1 out]
        n84 = for {
          tunnel: w366 -> [w370] mode=indexing
          tunnel: w365 -> [w374] mode=indexing
          tunnel: w348 -> [w372]
          tunnel: [w369] -> w363 mode=indexing
          n85 = Subtract(x=w374, y=w370) -> (x-y=w373:dbl)
          n86 = Multiply(x=w372, y=w373) -> (x*y=w371:dbl)
          n87 = Add(x=w370, y=w371) -> (x+y=w369:dbl)
        }
        n88 = Format Into String(format string="Calib Fraction %.4f; ", initial string=w347, w348) -> (resulting string=w345:string)  [unwired: 1 in, 1 out]
        n89 = call <vilib>:"General Polynomial Fit.vi"("Y"=w363, "polynomial order"=2, "X"=w364) -> ("Polynomial Coefficients"=w360:dbl[])  [unwired: 9 in, 3 out]
        n90 = Replace Array Subset(array=w359, new element=w360, index=0) -> (w358:dbl[])
      }
      frame "Single Hot wire" {
        n91 = Index Array(array=w383, index (col)=1) -> (element=w382:dbl[])  [unwired: 1 in]
        n92 = Index Array(array=w383, index (col)=0) -> (element=w381:dbl[])  [unwired: 1 in]
        n93 = Unbundle By Name(w398) -> ("Fraction"=w394:dbl)
        n94 = In Range and Coerce(upper limit=1.0, x=w394, lower limit=0.0) -> (coerced(x)=w380:dbl)  [unwired: 1 out]
        n95 = call "SingleWire_drift_correction_PN.vi"("calib consts. t1"=w387, "Tmeas (degC)"=w378, "variable n"=w377, "calib consts. t2"=w386, "{E_cal1}"=w382, "{U_cal1}"=w381, "time fraction"=w380, "wire diameter (mu.m)"=w376) -> ("[A, B, n]"=w379:dbl[])  [unwired: 1 in, 6 out]
        n96 = Build Array (concatenate)(w379, w378) -> (w388:dbl[])
        n97 = Format Into String(format string="Calib Fraction %.4f; ", initial string=w391, w380) -> (resulting string=w389:string)  [unwired: 1 in, 1 out]
        n98 = Replace Array Subset(array=w387, new element=w388, index=0) -> (w400:dbl[])
      }
      frame "Cross wire" {
        n99 = for {
          tunnel: w431 -> [w488]
          tunnel: w432 -> [w487]
          tunnel: [w486] -> w425 mode=indexing
          tunnel: [w485] -> w424 mode=indexing
          tunnel: i32[] [0, 1, 2, 9, 10, 12, 14, 15] -> [w484] mode=indexing
          n100 = Index Array(array=w488, index=w484) -> (element=w486:dbl)
          n101 = Index Array(array=w487, index=w484) -> (element=w485:dbl)
        }
        n102 = for {
          tunnel: i32[] [3, 4, 5, 9, 11, 13, 16, 17] -> [w483] mode=indexing
          tunnel: w432 -> [w482]
          tunnel: [w481] -> w417 mode=indexing
          tunnel: w431 -> [w480]
          tunnel: [w479] -> w418 mode=indexing
          n103 = Index Array(array=w480, index=w483) -> (element=w479:dbl)
          n104 = Index Array(array=w482, index=w483) -> (element=w481:dbl)
        }
        n105 = Index Array(array=w421, index (col)=1) -> (element=w423:dbl[])  [unwired: 1 in]
        n106 = Index Array(array=w421, index (col)=0) -> (element=w420:dbl[])  [unwired: 1 in]
        n107 = Index Array(array=w421, index (col)=2) -> (element=w419:dbl[])  [unwired: 1 in]
        n108 = Unbundle By Name(w445) -> ("Fraction"=w441:dbl)
        n109 = In Range and Coerce(upper limit=1.0, x=w441, lower limit=0.0) -> (coerced(x)=w416:dbl)  [unwired: 1 out]
        n110 = call "SingleWire_drift_correction_PN.vi"("calib consts. t1"=w425, "Tmeas (degC)"=w412, "variable n"=w413, "calib consts. t2"=w424, "{E_cal1}"=w423, "{U_cal1}"=w420, "time fraction"=w416, "wire diameter (mu.m)"=w411) -> ("[A, B, n]"=w415:dbl[])  [unwired: 1 in, 6 out]
        n111 = call "SingleWire_drift_correction_PN.vi"("calib consts. t1"=w418, "Tmeas (degC)"=w412, "variable n"=w413, "calib consts. t2"=w417, "{E_cal1}"=w419, "{U_cal1}"=w420, "time fraction"=w416, "wire diameter (mu.m)"=w411) -> ("[A, B, n]"=w414:dbl[])  [unwired: 1 in, 6 out]
        n112 = Replace Array Subset(array=w431, new element=w412, index=9) -> (w427:dbl[])
        n113 = Replace Array Subset(array=w427, new element=w415, index=0) -> (w426:dbl[])
        n114 = Replace Array Subset(array=w426, new element=w414, index=3) -> (w407:dbl[])
        n115 = Format Into String(format string="Calib Fraction %.4f; ", initial string=w438, w416) -> (resulting string=w436:string)  [unwired: 1 in, 1 out]
        n116 = case shown="False" w409 {
          tunnel: w410 -> [w454 _]
          tunnel: w408 -> [w448 _]
          tunnel: w407 -> [w453 _]
          tunnel: w406 -> [w452 _]
          tunnel: w405 -> [w451 _]
          tunnel: w404 -> [w450 _]
          tunnel: w403 -> [w449 _]
          frame False {
            n117 = case shown="\"Triangle mesh\", \"Polynomial surface\"" w448 {
              selector: w448 -> [w461 _ _]
              tunnel: w454 -> [w469 _ _]
              tunnel: w453 -> [w466 _ _]
              tunnel: w452 -> [w465 _ _]
              tunnel: w451 -> [w464 _ _]
              tunnel: w450 -> [w463 _ _]
              tunnel: w449 -> [w462 _ _]
              frame "Triangle mesh", "Polynomial surface" {
                n118 = Strip Path(path=w469) -> (stripped path=w458:path)  [unwired: 1 out]
                n119 = Build Path(base path=w458, name or relative path="XW_Map.txt") -> (appended path=w467:path)
                n120 = Build Path(base path=w458, name or relative path="XW_Map_CALPTS.txt") -> (appended path=w460:path)
                n121 = call "Does_file_exist_(simple).vi"("Pathname"=w467) -> ("exists?"=w456:bool)
                n122 = call "Does_file_exist_(simple).vi"("Pathname"=w460) -> ("exists?"=w457:bool)
                n123 = And(x=w456, y=w457) -> (x .and. y?=w455:bool)
                n124 = case shown="True" w455 {
                  tunnel: w467 -> [_ w476]
                  tunnel: w461 -> [_ w477]
                  tunnel: w466 -> [_ w475]
                  tunnel: w465 -> [_ w474]
                  tunnel: w464 -> [_ w473]
                  tunnel: w463 -> [_ w472]
                  tunnel: w462 -> [_ w471]
                  frame False {
                    n125 = global write "XW_Map_Global.vi" "Map method"(Map_method."Const. Psi_eff (std.)" ("Map method")) -> ()
                  }
                  frame True {
                    n126 = call "XW_Map_PreProc_wrapper_PN.vi"("Domain padding factor"=w471, "cap indicial sum to n"=w472, "XW_Calib_Map file path"=w476, "surface order (n)"=w473, "Apply calibration corrections"=w474, "Calib const"=w475, "Map method"=w477) -> ()  [unwired: 5 out]
                  }
                }
              }
              frame "Psi_eff = f(Umagn.)", "Psi_eff, k = f(Umagn.)" {
              }
              frame "Const. Psi_eff (std.)" {
                n127 = global write "XW_Map_Global.vi" "Map method"(Map_method."Const. Psi_eff (std.)" ("Map method")) -> ()
              }
            }
          }
          frame True {
          }
        }
      }
      frame "FFID Bkgnd correction method" {
        n128 = Strip Path(path=w494) -> (stripped path=w498:path)  [unwired: 1 out]
        n129 = Build Path(base path=w498, name or relative path="Background_History.xls") -> (appended path=w497:path)
        n130 = call "Does_file_exist_(simple).vi"("Pathname"=w497) -> ("exists?"=w496:bool)
        n131 = Select(t="Bkgnd info from table", s=w496, f="Bkgnd info from header") -> (s? t:f=w495:string)
      }
      frame "Bkgnd info from header" {
        n132 = stacked-sequence {
          seq-local: [w524 _ _ _] -> [_ _ w569 _]
          seq-local: [w536 _ _ _] -> [_ _ w567 _]
          seq-local: [w531 _ _ _] -> [_ _ w566 _]
          seq-local: [_ w559 _ _] -> [_ _ w565 _]
          seq-local: [_ _ w564 _] -> [_ _ _ w665]
          tunnel: w523 -> [w538 w558 _ _]
          tunnel: w522 -> [_ _ w568 _]
          tunnel: w521 -> [_ w554 _ _]
          tunnel: [_ w558 _ _] -> w520
          tunnel: w519 -> [_ w557 _ _]
          tunnel: [_ w557 _ _] -> w518
          tunnel: [_ w556 _ _] -> w517
          tunnel: w516 -> [_ w556 _ _]
          tunnel: w515 -> [_ _ _ w675]
          tunnel: [_ _ _ w672] -> w514
          tunnel: [_ w555 _ _] -> w513
          tunnel: w512 -> [_ w555 _ _]
          tunnel: [_ _ _ "Add FFID Bkgnd Values"] -> w511
          tunnel: [_ _ _ TRUE] -> w510
          tunnel: [_ w554 _ _] -> w509
          tunnel: [_ _ _ w667] -> w508
          tunnel: w507 -> [_ _ _ w666]
          frame #0 {
            n133 = Concatenate Strings("Calibration To be Used" ("Input Element"), "\t") -> (w540:string)
            n134 = Match Pattern(string=w538, regular expression=w540) -> (before substring=w545:string, match substring=w551:string, after substring=w552:string)  [unwired: 2 out]
            n135 = Reverse String(1:w545) -> (0:w546:string)
            n136 = Match Pattern(string=w546, regular expression="[*][*][*][*][*][*][*][*][*][*][*][*][*][\t][*][*][*][*][*][*][*][*][*][*][*][*][*][\t][*][*][*][*][*][*][*][*][*][*][*][*][*][\t][*][*][*][*]" ("String")) -> (before substring=w544:string)  [unwired: 4 out]
            n137 = Reverse String(1:w544) -> (0:w543:string)
            n138 = call "Split_at_return.vi"("String"=w543) -> ("after substring"=w542:string)  [unwired: 1 in, 3 out]
            n139 = call "String_to_Ch_names.vi"("Spreadsheet string"=w542) -> ("Ch names"=w536:string[], "String After names"=w550:string)  [unwired: 2 out]
            n140 = Concatenate Strings(w550, w551, w552) -> (w553:string)
            n141 = Search 1D Array(1D array=w536, element="FF:1:Bkgnd Volts") -> (index of element=w530:i32)  [unwired: 1 out]
            n142 = Spreadsheet String To Array(format string="%s", spreadsheet string=w553, array type (2D Dbl)=string[][] []) -> (array=w531:string[][])  [unwired: 1 out]
            "Header info" <- w531
            n143 = Index Array(array=w531, index (col)=0 ("disabled index (col)")) -> (element=w533:string[])  [unwired: 1 in]
            n144 = Search 1D Array(1D array=w533, element="Calibration After Meas") -> (index of element=w532:i32)  [unwired: 1 out]
            n145 = Index Array(array=w531, index (row)=w532, index (col)=w530) -> (element=w529:string)
            n146 = Match Pattern(string=w529, regular expression="_Place_Holder") -> (offset past match=w527:i32)  [unwired: 4 out]
            n147 = Less Than 0?(x=w527) -> (x < 0?=w525:bool)
            n148 = Greater Or Equal To 0?(x=w530) -> (x >= 0?=w526:bool)
            n149 = And(x=w526, y=w525) -> (x .and. y?=w524:bool)
          }
          frame #1 {
            n150 = Unbundle By Name(w554) -> ("Meas start time"=w563:dbl, "Meas end time"=w562:dbl)
            n151 = Add(x=w563, y=w562) -> (x+y=w561:dbl)
            n152 = Divide(x=w561, y=2.0) -> (x/y=w559:dbl)
          }
          frame #2 {
            n153 = case shown="False" w569 {
              tunnel: w568 -> [w585 w639]
              tunnel: w567 -> [w572 w629]
              tunnel: w566 -> [w574 w630]
              tunnel: w565 -> [w571 _]
              tunnel: [w570 w622] -> w564
              frame True {
                n154 = Decimal String To Number(string=w585) -> (number=w584:i32)  [unwired: 3 out]
                n155 = Index Array(array=w574, index (col)=0 ("disabled index (col)")) -> (element=w579:string[])  [unwired: 1 in]
                n156 = Number To Decimal String(number=w584) -> (decimal integer string=w583:string)  [unwired: 1 out]
                n157 = Search 1D Array(1D array=w579, element="Calibration Before Meas") -> (index of element=w577:i32)  [unwired: 1 out]
                n158 = Search 1D Array(1D array=w579, element="Calibration After Meas") -> (index of element=w575:i32)  [unwired: 1 out]
                n159 = Index Array(array=w574, index (row)=w577) -> (element=w576:string[])  [unwired: 1 in]
                n160 = Index Array(array=w574, index (row)=w575) -> (element=w573:string[])  [unwired: 1 in]
                n161 = for {
                  tunnel: w583 -> [w601]
                  tunnel: string[] ["Bkgnd Time", "Bkgnd Volts", "Bkgnd Variance"] ("appended array") -> [w600] mode=indexing
                  tunnel: w576 -> [w599]
                  tunnel: w573 -> [w597]
                  tunnel: w572 -> [w595]
                  tunnel: w571 -> [w593]
                  shift-right: [w587] -> _
                  shift-left: _ -> [w588]
                  tunnel: [w586] -> w570 mode=indexing
                  i -> [w594]
                  # "After"
                  # "Before"
                  n162 = Concatenate Strings("FF:", w601, ":" ("Substring"), w600) -> (w602:string)
                  n163 = Search 1D Array(1D array=w595, element=w602) -> (index of element=w598:i32)  [unwired: 1 out]
                  n164 = Index Array(array=w599, index=w598) -> (element=w592:string)
                  n165 = Index Array(array=w597, index=w598) -> (element=w591:string)
                  n166 = call "String_2_Number.vi"("Value"=w592) -> ("Numeric"=w590:dbl)
                  n167 = call "String_2_Number.vi"("Value"=w591) -> ("Numeric"=w589:dbl)
                  n168 = case shown="1, Default" w594 {
                    tunnel: w593 -> [w609 _]
                    tunnel: w590 -> [w607 w612]
                    tunnel: w589 -> [w608 w615]
                    tunnel: [w604 w611] -> w586
                    tunnel: w588 -> [_ w610]
                    tunnel: [w604 w610] -> w587
                    frame 0 {
                      n169 = Subtract(x=w609, y=w607) -> (x-y=w605:dbl)
                      n170 = Subtract(x=w608, y=w607) -> (x-y=w606:dbl)
                      n171 = Divide(x=w605, y=w606) -> (x/y=w604:dbl)
                    }
                    frame 1, Default {
                      n172 = Subtract(x=w615, y=w612) -> (x-y=w614:dbl)
                      n173 = Multiply(x=w610, y=w614) -> (x*y=w613:dbl)
                      n174 = Add(x=w613, y=w612) -> (x+y=w611:dbl)
                    }
                  }
                }
              }
              frame False {
                n175 = Decimal String To Number(string=w639) -> (number=w638:i32)  [unwired: 3 out]
                n176 = Index Array(array=w630, index (col)=0 ("disabled index (col)")) -> (element=w633:string[])  [unwired: 1 in]
                n177 = Number To Decimal String(number=w638) -> (decimal integer string=w637:string)  [unwired: 1 out]
                n178 = Search 1D Array(1D array=w633, element="Calibration To be Used") -> (index of element=w632:i32)  [unwired: 1 out]
                n179 = Index Array(array=w630, index (row)=w632) -> (element=w631:string[])  [unwired: 1 in]
                n180 = for {
                  tunnel: w637 -> [w660]
                  tunnel: string[] ["Coeff A", "Coeff B", "Coeff C", "Bkgnd", "Bkgnd Variance"] ("appended array") -> [w659] mode=indexing
                  tunnel: w631 -> [w658]
                  tunnel: w629 -> [w656]
                  tunnel: [w654] -> w618 mode=indexing
                  tunnel: [w653] -> w621 mode=indexing
                  n181 = Concatenate Strings("FF:", w660, ":" ("Substring"), w659) -> (w661:string)
                  n182 = Search 1D Array(1D array=w656, element=w661) -> (index of element=w653:i32)  [unwired: 1 out]
                  n183 = Index Array(array=w658, index=w653) -> (element=w655:string)
                  n184 = call "String_2_Number.vi"("Value"=w655) -> ("Numeric"=w654:dbl)
                }
                n185 = Index Array(array=w618, index=3 ("length")) -> (element=w627:dbl)
                n186 = Index Array(array=w618, index=4) -> (element=w624:dbl)
                n187 = Index Array(array=w621, index=2) -> (element=w619:i32)
                n188 = Less Than 0?(x=w619) -> (x < 0?=w617:bool)
                n189 = case shown="True" w617 {
                  tunnel: w618 -> [w641 w647]
                  tunnel: [w640 w643] -> w616
                  frame False {
                    n190 = Array Subset(array=w641, length=3) -> (w640:dbl[])  [unwired: 1 in]
                  }
                  frame True {
                    n191 = Index Array(array=w647, index=1) -> (element=w651:dbl)
                    n192 = Index Array(array=w647, index=0) -> (element=w650:dbl)
                    n193 = Reciprocal(x=w651) -> (1/x=w645:dbl)
                    n194 = Divide(x=w650, y=w651) -> (x/y=w652:dbl)
                    n195 = Negate(x=w652) -> (-x=w646:dbl)
                    n196 = Build Array(w646, w645, 0.0 ("element")) -> (w643:dbl[])
                  }
                }
                n197 = call "Polybackwards.vi"("Coefficients"=w616, "Y input"=w627) -> ("X output"=w625:dbl)  [unwired: 1 out]
                n198 = Build Array(0.0 ("element"), w625, w624) -> (w622:dbl[])
              }
            }
          }
          frame #3 {
            n199 = Index Array(array=w665, index=1) -> (element=w677:dbl)
            n200 = Index Array(array=w665, index=2) -> (element=w673:dbl)
            n201 = Build Array(w677) -> (w681:dbl[])
            n202 = Index Array(array=w665, index=0) -> (element=w668:dbl)
            n203 = call "2nd_order_Poly_convert.vi"("Calib constants"=w675, "Voltage"=w681) -> ("Eng Values"=w680:dbl[])  [unwired: 4 out]
            n204 = Not A Number/Path/Refnum?(number/path/refnum=w665) -> (NaN/Path/Refnum?=w664:bool[])
            n205 = Or Array Elements(Boolean array=w664) -> (logical OR=w663:bool)
            n206 = Index Array(array=w680, index=0) -> (element=w674:dbl)
            n207 = case shown="False" w663 {
              tunnel: w675 -> [w694 w695]
              tunnel: w674 -> [w692 _]
              tunnel: w673 -> [w689 _]
              tunnel: [w688 w695] -> w672
              tunnel: w668 -> [w686 _]
              tunnel: [w683 w696] -> w667
              tunnel: w666 -> [w682 w696]
              frame False {
                n208 = Equal To 0?(x=w686) -> (x = 0?=w685:bool)
                n209 = Replace Array Subset(array=w694, new element=w692, index=3) -> (w691:dbl[])
                n210 = Format Into String(format string="Bkgnd Fraction %.4f; ", initial string=w682, w686) -> (resulting string=w684:string)  [unwired: 1 in, 1 out]
                n211 = Replace Array Subset(array=w691, new element=w689, index=4) -> (w688:dbl[])
                n212 = Select(t=w682, s=w685, f=w684) -> (s? t:f=w683:string)
              }
              frame True {
              }
            }
          }
        }
      }
      frame "Bkgnd info from table" {
        n213 = stacked-sequence {
          seq-local: [w716 _] -> [_ w758]
          seq-local: [_ w772] -> [_ _]
          seq-local: [w717 _] -> [_ w773]
          seq-local: [w715 _] -> [_ w750]
          tunnel: w714 -> [_ w781]
          tunnel: w713 -> [_ w776]
          tunnel: w712 -> [_ w777]
          tunnel: [_ w781] -> w711
          tunnel: w710 -> [_ w780]
          tunnel: [_ w780] -> w709
          tunnel: [_ w779] -> w708
          tunnel: w707 -> [_ w779]
          tunnel: w706 -> [_ w764]
          tunnel: [_ w754] -> w705
          tunnel: [_ w778] -> w704
          tunnel: w703 -> [_ w778]
          tunnel: [_ "Add FFID Bkgnd Values"] -> w702
          tunnel: [_ TRUE] -> w701
          tunnel: [_ w777] -> w700
          tunnel: w699 -> [_ w760]
          tunnel: [_ w759] -> w698
          frame #0 {
            n214 = while {
              shift-right: [w726] -> _
              shift-left: _ -> [w727]
              shift-right: [w724] -> w717
              shift-left: _ -> [w722]
              shift-right: [w723] -> w716
              shift-left: _ -> [w721]
              shift-right: [w719] -> w715
              shift-left: _ -> [w718]
              stop <- TRUE stop-if-true
              n215 = global read "Meas_global.vi" "Raw data file"() -> (w730:path)
              n216 = Strip Path(path=w730) -> (stripped path=w728:path)  [unwired: 1 out]
              n217 = Build Path(base path=w728, name or relative path="Background_History.xls") -> (appended path=w726:path)
              n218 = Equal?(x=w726, y=w727) -> (x = y?=w725:bool)
              n219 = case shown="False" w725 {
                tunnel: w726 -> [w744 _]
                tunnel: [w737 w747] -> w724
                tunnel: [w734 w746] -> w723
                tunnel: w722 -> [_ w747]
                tunnel: w721 -> [_ w746]
                tunnel: [w731 w745] -> w719
                tunnel: w718 -> [_ w745]
                frame False {
                  n220 = call "Read_File_Simple.vi"("Filename"=w744) -> ("string"=w743:string)  [unwired: 2 in, 7 out]
                  n221 = call "String_to_Ch_names.vi"("Spreadsheet string"=w743) -> ("Ch names"=w733:string[], "String After names"=w740:string)  [unwired: 2 out]
                  n222 = Spreadsheet String To Array(format string="%s", spreadsheet string=w740, array type (2D Dbl)=string[][] []) -> (array=w736:string[][])  [unwired: 1 out]
                  n223 = Search 1D Array(1D array=w733, element="Seconds:since:1st Jan") -> (index of element=w735:i32)  [unwired: 1 out]
                  n224 = Increment(x=w735) -> (x+1=w732:i32)
                  n225 = Index Array(array=w736, index (col)=w735) -> (element=w738:string[])  [unwired: 1 in]
                  n226 = Array Subset(array=w736, index (col)=w732) -> (w734:string[][])  [unwired: 3 in]
                  n227 = call "String_2_Number_array.vi"("Input String"=w738) -> ("Values"=w737:dbl[])
                  n228 = Array Subset(array=w733, index=w732) -> (w731:string[])  [unwired: 1 in]
                }
                frame True {
                }
              }
            }
          }
          frame #1 {
            n229 = Unbundle By Name(w777) -> ("Meas start time"=w785:dbl, "Meas end time"=w784:dbl)
            n230 = Decimal String To Number(string=w776) -> (number=w752:i32)  [unwired: 3 out]
            n231 = Format Into String(format string="FF:%d:Bkgnd c^2", w752) -> (resulting string=w751:string)  [unwired: 2 in, 1 out]
            n232 = Search 1D Array(1D array=w750, element=w751) -> (index of element=w749:i32)  [unwired: 1 in]
            n233 = Decrement(x=w752) -> (x-1=w775:i32)
            n234 = Add(x=w785, y=w784) -> (x+y=w783:dbl)
            n235 = Divide(x=w783, y=2.0) -> (x/y=w772:dbl)
            n236 = Index Array(array=w758, index (col)=w775) -> (element=w774:string[])  [unwired: 1 in]
            n237 = Threshold 1D Array(2:w772, 3:w773) -> (0:w757:dbl)  [unwired: 1 out]
            n238 = case shown="1, Default" w749 {
              tunnel: w758 -> [_ w794]
              tunnel: w757 -> [_ w789]
              tunnel: [0.22 w791] -> w753
              tunnel: w749 -> [_ w790]
              frame -1 {
              }
              frame 1, Default {
                n239 = Index Array(array=w794, index (col)=w790) -> (element=w793:string[])  [unwired: 1 in]
                n240 = call "String_2_Number_array.vi"("Input String"=w793) -> ("Values"=w792:dbl[])
                n241 = Interpolate 1D Array(1:w789, 2:w792) -> (0:w791:dbl)
              }
            }
            n242 = for {
              tunnel: w774 -> [w787] mode=indexing
              tunnel: [w786] -> w771 mode=indexing
              n243 = call "String_2_Number.vi"("Value"=w787) -> ("Numeric"=w786:dbl)
            }
            n244 = Interpolate 1D Array(1:w757, 2:w771) -> (0:w763:dbl)
            n245 = Build Array(w763) -> (w767:dbl[])
            n246 = Format Into String(format string="Bkgnd Index %.2f; ", initial string=w760, w757) -> (resulting string=w759:string)  [unwired: 1 in, 1 out]
            n247 = call "2nd_order_Poly_convert.vi"("Calib constants"=w764, "Voltage"=w767) -> ("Eng Values"=w766:dbl[])  [unwired: 4 out]
            n248 = Index Array(array=w766, index=0) -> (element=w762:dbl)
            n249 = Replace Array Subset(array=w764, new element=w762, index=3) -> (w755:dbl[])
            n250 = Replace Array Subset(array=w755, new element=w753, index=4) -> (w754:dbl[])
          }
        }
      }
      frame "Add FFID Bkgnd Values" {
        n251 = global read "Plug_in_data_global.vi" "FFID Bkgnd Values"() -> (w799:dbl[])
        n252 = Array Size(array=w799) -> (size(s)=w803:i32)
        n253 = Greater Than 0?(x=w803) -> (x > 0?=w802:bool)
        n254 = case shown="True" w802 {
          tunnel: w801 -> [w811 w825]
          tunnel: [w811 w824] -> w800
          tunnel: w799 -> [_ w815]
          tunnel: w798 -> [w810 w818]
          tunnel: [w810 w812] -> w797
          frame False {
          }
          frame True {
            # "20 blocks of 3 sec bkgnd"
            n255 = Index Array(array=w815, index=1) -> (element=w817:dbl)
            n256 = Index Array(array=w815, index=0) -> (element=w822:dbl)
            n257 = Index Array(array=w815, index=2) -> (element=w814:dbl)
            n258 = Array Subset(array=w815, index=3) -> (w820:dbl[])  [unwired: 1 in]
            n259 = global write "Plug_in_data_global.vi" "FFID Bkgnd Values"(w820) -> ()
            n260 = Replace Array Subset(array=w825, new element=w822, index=3) -> (w824:dbl[])
            n261 = Format Into String(format string="%d blocks of %d Sec Bkgnd; ", initial string=w818, w817, w814) -> (resulting string=w812:string)  [unwired: 1 in, 1 out]
          }
        }
      }
      frame "Add Drift Info" {
        n262 = call "Get_Characters_from_string.vi"("Show Dialog?"=FALSE, "Input string"=w838, "Variable name"="Percentage Drift till Next calibration") -> ("Status"=w845:enum16{"Char in string", "Char not in string"}, "Value"=w846:string)
        n263 = Empty String/Path?(string/path=w834) -> (empty?=w833:bool)
        n264 = case shown="True" w833 {
          tunnel: w834 -> [w879 _]
          tunnel: w828 -> [w877 w881]
          tunnel: [w874 w881] -> w827
          frame False {
            n265 = Unbundle By Name(w877) -> ("Extra Titles"=w878:string[], "Extra Values"=w880:string[])
            n266 = Build Array (concatenate)(w880, w879) -> (w875:string[])
            n267 = Build Array (concatenate)(w878, "Correction:Info" ("string")) -> (w876:string[])
            n268 = Bundle By Name(cluster=w877, "Extra Titles"=w876, "Extra Values"=w875) -> (w874:T1)
          }
          frame True {
          }
        }
        n269 = case shown="\"Char not in string\"" w845 {
          tunnel: [w888 nan ("Value")] -> w837
          tunnel: w846 -> [w884 _]
          frame "Char in string" {
            n270 = Match Pattern(string=w884, regular expression="Drift_Place_Holder") -> (offset past match=w886:i32)  [unwired: 4 out]
            n271 = Greater Than 0?(x=w886) -> (x > 0?=w885:bool)
            n272 = case shown="False" w885 {
              tunnel: [w889 nan ("Value")] -> w888
              tunnel: w884 -> [w890 _]
              frame False {
                n273 = call "String_2_Number.vi"("Value"=w890) -> ("Numeric"=w889:dbl)
              }
              frame True {
              }
            }
          }
          frame "Char not in string" {
          }
        }
        n274 = call "Get_value_from_string.vi"("Show Dialog?"=FALSE, "Input string"=w838, "Variable name"="Minutes Until Next calibration") -> ("Status"=w841:enum16{"Char in string", "Char not in string"}, "Value"=w842:dbl)
        n275 = Array Size(array=w847) -> (size(s)=w848:i32)
        n276 = case shown="\"Char not in string\"" w841 {
          tunnel: [w882 nan ("Value")] -> w836
          tunnel: w842 -> [w882 _]
          frame "Char in string" {
          }
          frame "Char not in string" {
          }
        }
        n277 = Subtract(x=18, y=w848) -> (x-y=w850:i32)
        n278 = Initialize Array(0.0 ("Element Data"), w850) -> (w852:dbl[])
        n279 = Build Array (concatenate)(w847, w852, w837, w836) -> (w832:dbl[])
        n280 = case shown="False" w830 {
          tunnel: w831 -> [w859 _]
          tunnel: w829 -> [w858 _]
          frame False {
            n281 = case shown="\"Psi_eff = f(Umagn.)\", \"Psi_eff, k = f(Umagn.)\"" w858 {
              selector: w858 -> [_ w866 _]
              tunnel: w859 -> [_ w869 _]
              frame "Triangle mesh", "Polynomial surface" {
              }
              frame "Psi_eff = f(Umagn.)", "Psi_eff, k = f(Umagn.)" {
                n282 = Strip Path(path=w869) -> (stripped path=w864:path)  [unwired: 1 out]
                n283 = Build Path(base path=w864, name or relative path="XW_Map.txt") -> (appended path=w867:path)
                n284 = Build Path(base path=w864, name or relative path="XW_Map_CALPTS.txt") -> (appended path=w863:path)
                n285 = call "Does_file_exist_(simple).vi"("Pathname"=w867) -> ("exists?"=w862:bool)
                n286 = call "Does_file_exist_(simple).vi"("Pathname"=w863) -> ("exists?"=w861:bool)
                n287 = And(x=w862, y=w861) -> (x .and. y?=w860:bool)
                n288 = case shown="True" w860 {
                  tunnel: w866 -> [_ w871]
                  frame False {
                    n289 = global write "XW_Map_Global.vi" "Map method"(Map_method."Const. Psi_eff (std.)" ("Map method")) -> ()
                  }
                  frame True {
                    n290 = call "XW_Higher_order_Psi_k_PreProc_PN.vi"("Map method"=w871) -> ()  [unwired: 1 in, 1 out]
                  }
                }
              }
              frame "Const. Psi_eff (std.)" {
                n291 = global write "XW_Map_Global.vi" "Map method"(Map_method."Const. Psi_eff (std.)" ("Map method")) -> ()
              }
            }
          }
          frame True {
          }
        }
      }
    }
  }
  "Calib Coeff" <- w21
  "Analysis Info cluster  Out" <- w5
